vi "SelPO.vi"() -> (2 "MainPOSel":bool, 3 "AddPOSel":bool)   [LabVIEW 2017]
panel:
  in  "AddPO":bool
  in  "MainPO":bool
  # "Внимание! Масштабирование экрана должно быть \nустановлено 100% в \"Настройка экрана\".\nИспользование ПО с другим масштабом недопустимо!"
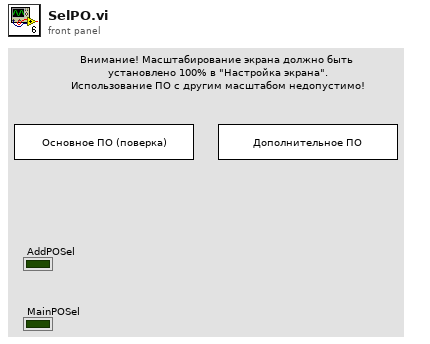
[diagram p1: front panel]
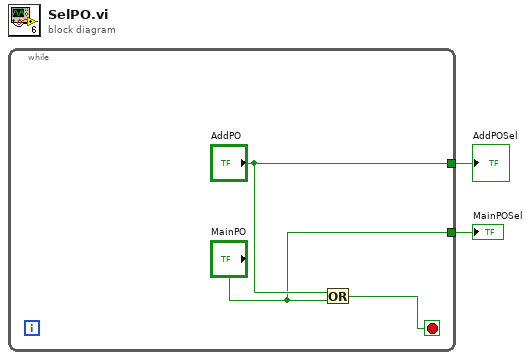
[diagram p0: block diagram]
diagram:
  n1 = while {
    tunnel: ["AddPO"] -> w2
    tunnel: ["MainPO"] -> w1
    stop <- w5 stop-if-true
    n2 = Or(x="AddPO", y="MainPO") -> (x .or. y?=w5:bool)
  }
  "AddPOSel" <- w2
  "MainPOSel" <- w1
